vi "RunVI.vi"(8 "VI引用句柄":refnum<vi>, 10 "Run?(Default Abort)":bool, 11 "Front Panel Window:Open":bool) -> ()   [LabVIEW 2011]
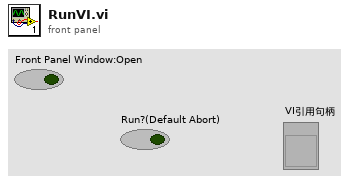
[diagram p1: front panel]
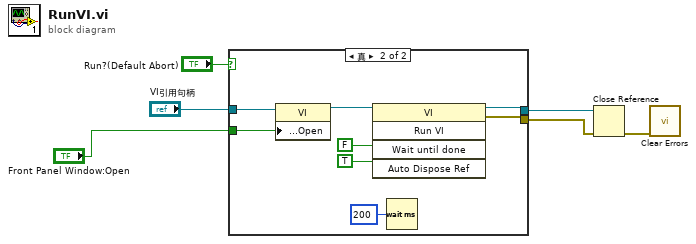
[diagram p0: block diagram]
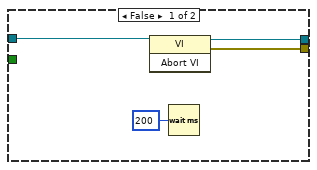
[diagram p2: hidden frame]
diagram:
  n1 = case shown="真" "Run?(Default Abort)" {
    tunnel: [w10 w16] -> w6
    tunnel: [w9 w15] -> w5
    tunnel: "VI引用句柄" -> [w7 w13]
    tunnel: "Front Panel Window:Open" -> [_ w11]
    frame False {
      n2 = invoke class="VI" method="Abort VI"(reference=w7) -> (reference out=w10:refnum<vi>, error out=w9:errorcluster)  [unwired: 2 in, 1 out]
      n3 = Wait (ms)(milliseconds to wait=u32 200) -> ()  [unwired: 1 out]
    }
    frame True {
      n4 = property class="VI"(reference=w13, "Front Panel.Open"=w11) -> (reference out=w12:refnum<vi>)  [unwired: 1 in, 1 out]
      n5 = invoke class="VI" method="Run VI"(reference=w12, "Wait until done"=FALSE ("Wait Until Done"), "Auto Dispose Ref"=TRUE ("Auto Dispose Reference")) -> (reference out=w16:refnum<vi>, error out=w15:errorcluster)  [unwired: 2 in, 3 out]
      n6 = Wait (ms)(milliseconds to wait=u32 200) -> ()  [unwired: 1 out]
    }
  }
  n7 = Close Reference(reference=w6, error in (no error)=w5) -> (error out=w3:errorcluster)
  n8 = call <vilib>:"Clear Errors.vi"("error in (no error)"=w3) -> ()  [unwired: 6 in, 1 out]
